vi "ZCAN_Filter(DTU).vi"(7 "error in (no error)":errorcluster caption="错误输入（无错误）", 9 "can_index":u32, 10 "device_handle":u32) -> (0 "error out":errorcluster caption="错误输出")   [LabVIEW 2013]
doc: "设置滤波，最多设置50条\n在SubVI内部设置，可根据项目实际需求修改\n在Init 初始化之后， Start 之前使用\n\n适用型号：USBCANFD-100U、USBCANFD-200U、USBCANFD-MINI、\nPCI-5010-U、PCI-5020-U、USBCAN-E-U、USBCAN-2E-U、CANalyst-II+、\nUSBCAN-4E-U"
panel:
  # "在后面板添加滤波表格"
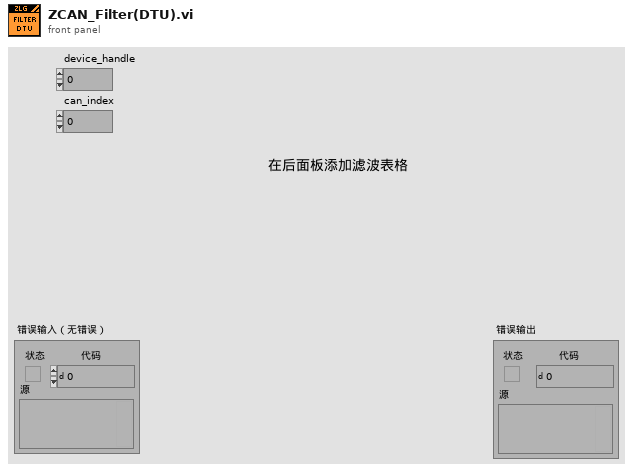
[diagram p1: front panel]
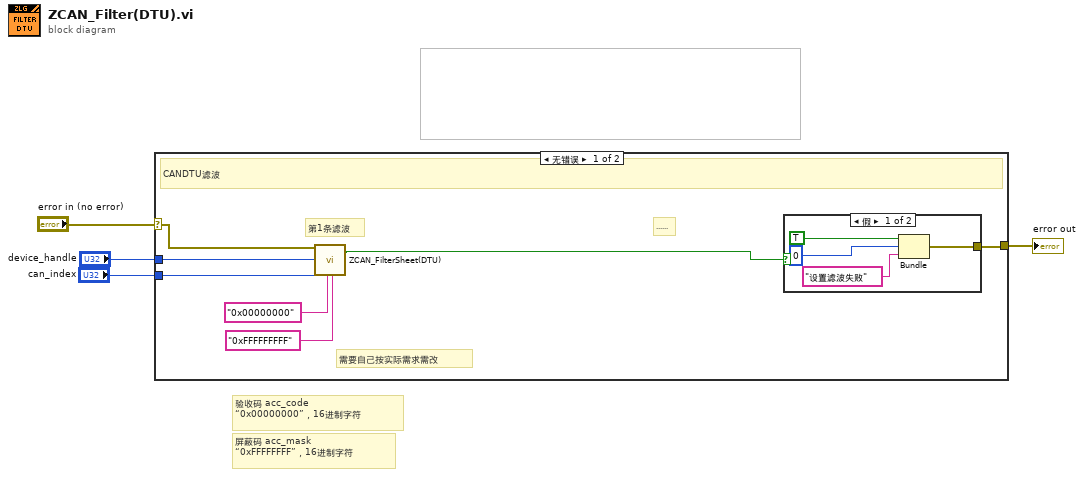
[diagram p0: block diagram]
diagram:
  # "屏蔽码\tacc_mask\t\n“0xFFFFFFFF”，16进制字符"
  # "验收码\tacc_code\t\n“0x00000000”，16进制字符"
  n1 = case shown="无错误" "error in (no error)" {
    selector: "error in (no error)" -> [w10 w16]
    tunnel: [w11 w16] -> w3
    tunnel: "device_handle" -> [w9 _]
    tunnel: "can_index" -> [w8 _]
    frame No Error {
      # "需要自己按实际需求需改"
      # "......"
      # "第1条滤波"
      # "CANDTU滤波"
      n2 = call "ZCAN_FilterSheet(DTU).vi"("error in (no error)"=w10, "can_index_handle"=w9, "can_index"=w8, "acc_code"="0x00000000" ("filter_start"), "acc_mask"="0xFFFFFFFFF" ("filter_end")) -> ("success?"=w5:bool)  [unwired: 11 in, 3 out]
      n3 = case shown="假" w5 {
        tunnel: [w12 _] -> w11
        frame False {
          n4 = Bundle("status"=TRUE, "code"=0, "消息"="设置滤波失败") -> (w12:cluster{"status":bool, "code":i32, "消息":string})  [unwired: 1 in]
        }
        frame True {
        }
      }
    }
    frame Error {
    }
  }
  "error out" <- w3
